vi "BRig_dataExp_Cue2_CueProb.vi"() -> (2 "output_Cue2_CueProb":i32)   [LabVIEW 2014]
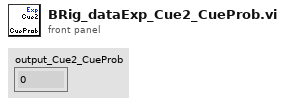
[diagram p1: front panel]
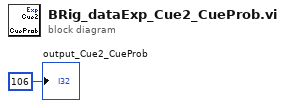
[diagram p0: block diagram]
diagram:
  "output_Cue2_CueProb" <- 106 ("output_iBlock")
